vi "Read tag selects.vi"(8 "error in (no error)":errorcluster, 11 "tag select module runtime in":refnum<class "tag select module runtime.lvclass">) -> (0 "error out":errorcluster, 2 "tag select":T1[](array[typedef]), 3 "tag select module runtime out":refnum<class "tag select module runtime.lvclass">)   [LabVIEW 2013, in "tag select module runtime.lvclass"]
uses:
  tag select module runtime.lvclass
  runtime tag select configuration.ctl
  <vilib>/NI/Tag Bus/tag/Data Type.ctl
  tag select module runtime.lvclass/tag select module runtime.ctl
  <vilib>/NI/Tag Bus/tag/tag descriptor.lvclass
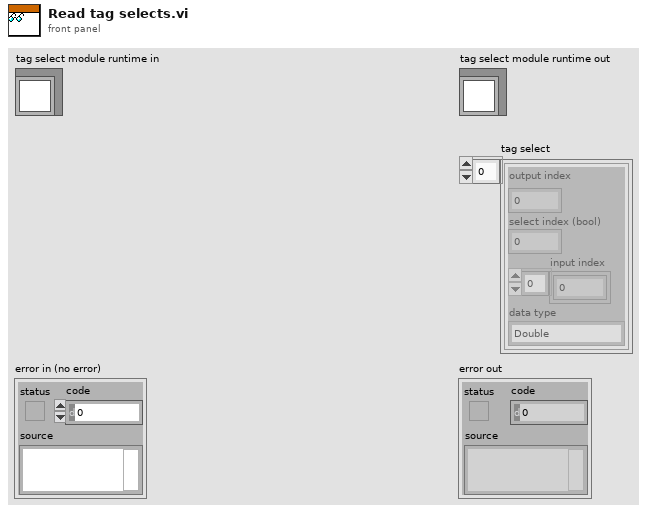
[diagram p1: front panel]
types:
  T1 = typedef "tag select module runtime.lvclass/runtime tag select configuration.ctl" = cluster{"output index":i32, "select index (bool)":i32, "input index":i32[], "data type":T2}
  T2 = typedef "tag bus.lvlib/tag descriptor.lvclass/Data Type.ctl" = enum16{"Double", "Single", "I64", "I32", "I16", "I8", "U64", "U32", "U16", "U8", "Boolean", "String", "Array of Double", "Array of Single", "Array of I64", "Array of I32", "Array of I16", "Array of I8", "Array of U64", "Array of U32", "Array of U16", "Array of U8", "Array of Boolean", "Array of String"}
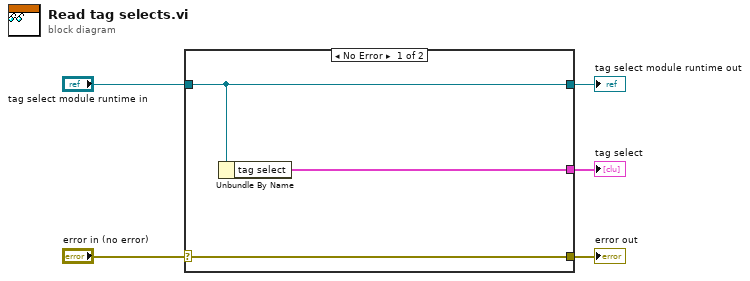
[diagram p0: block diagram]
diagram:
  n1 = case shown="No Error" "error in (no error)" {
    selector: "error in (no error)" -> [w8 w9]
    tunnel: [w8 w9] -> w4
    tunnel: [w7 w10] -> w2
    tunnel: "tag select module runtime in" -> [w7 w10]
    tunnel: [w6 _] -> w1
    frame No Error {
      n2 = Unbundle By Name(w7) -> ("tag select"=w6:T1[])
    }
    frame Error {
    }
  }
  "error out" <- w4
  "tag select module runtime out" <- w2
  "tag select" <- w1
